vi "Create - Boolean Array.vi"(6 "timestamp in":timestamp, 8 "error in (no error)":errorcluster, 10 "value in":bool[](array[boolean])) -> (0 "error out":errorcluster, 3 "NT Scalar out":refnum<class "NT Scalar.lvclass">)   [LabVIEW 2020, in "PV Access.lvlib" / "PV Data.lvlib" / "NT Scalar.lvclass"]
uses:
  NT Scalar.lvclass
  NT Scalar.lvclass/NT Scalar.ctl
  3af84381-6f09-4a7d-a0f8-b098e3cc6b73.vi
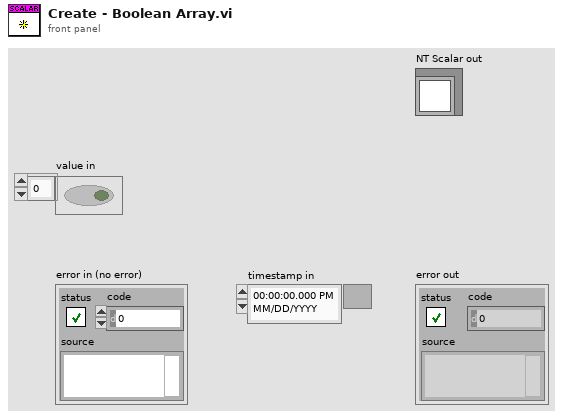
[diagram p1: front panel]
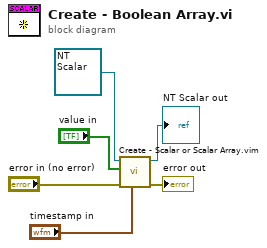
[diagram p0: block diagram]
diagram:
  n1 = call "Create - Scalar or Scalar Array.vim"("time stamp"="timestamp in", "error in (no error)"="error in (no error)", "value"="value in", "NT Scalar (Numeric) in"=refnum<class "NT Scalar.lvclass"> refnum ("NT Scalar in")) -> ("error out"=→"error out":errorcluster, "NT Scalar (Numeric) out"=→"NT Scalar out":refnum<class "NT Scalar.lvclass">)  [unwired: 6 in]
